vi "multi-graph-example-events.-simplevi.vi"() -> ()   [LabVIEW 2017]
panel:
  out "cycle #":i32
  in  "LSI-U CH labels":string[](array[string])
  out "labels S1":string[](array[string])
  in  "log/linear":bool
  in  "stop":bool
  out "Graph1 (4-10K)":cluster{timestamp[], dbl[]}[](graph)
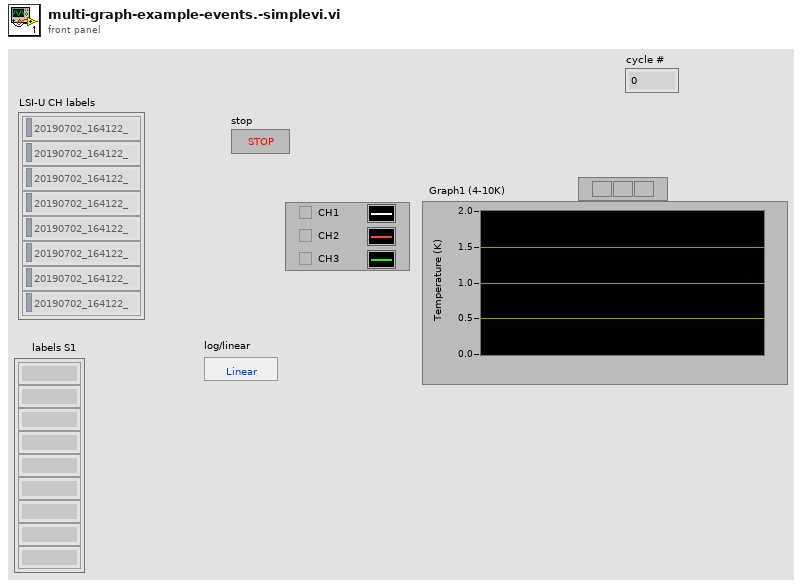
[diagram p1: front panel]
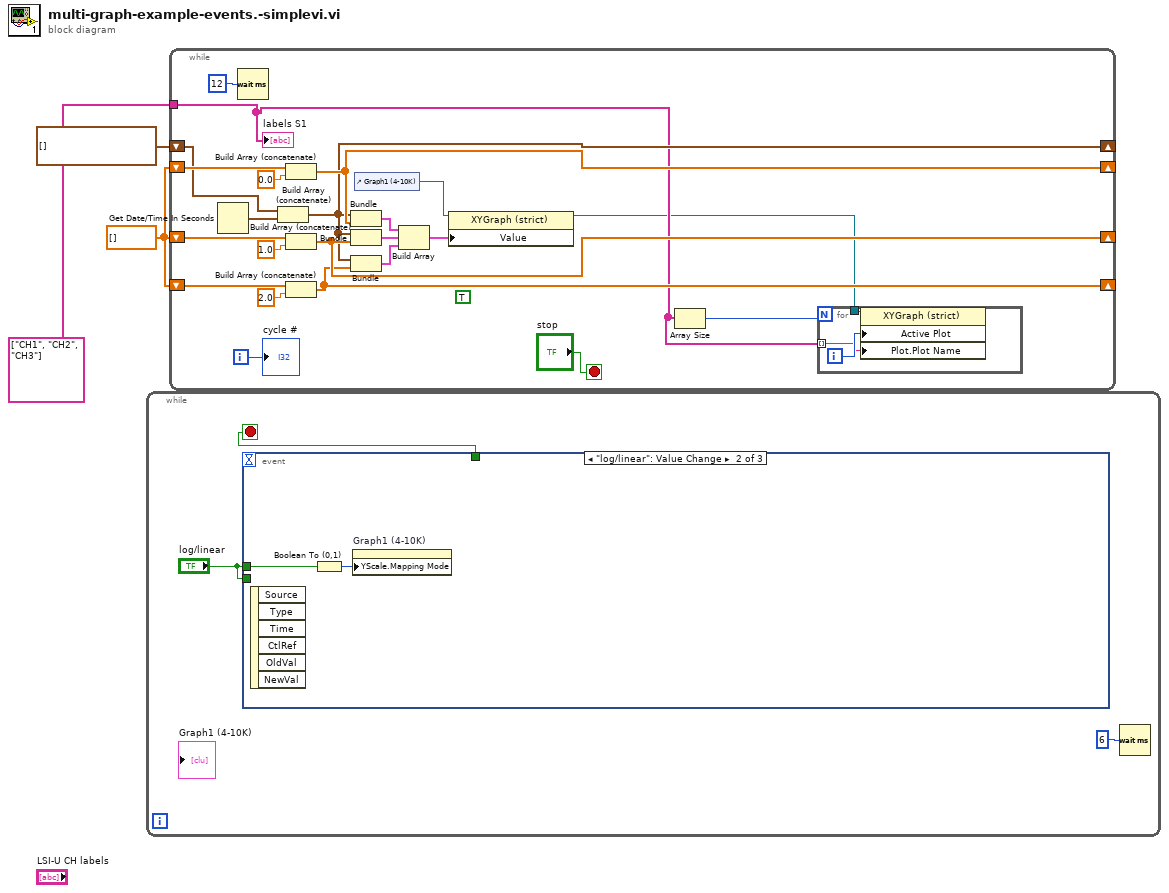
[diagram p0: block diagram]
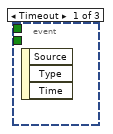
[diagram p2: hidden frame]
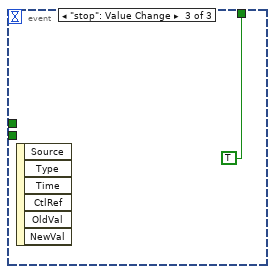
[diagram p3: hidden frame]
diagram:
  w2 = dbl[] []
  n1 = while {
    stop <- w4 stop-if-true
    n2 = event shown="[1] \"log/linear\": Value Change" {
      selector: _ -> [_ _ _]
      dyn-events: _ -> [_ _ _]
      timeout: _ -> [_ _ _]
      tunnel: "log/linear" -> [_ _ _]
      tunnel: "log/linear" -> [_ w7 _]
      tunnel: [_ _ TRUE] -> w4
      event Timeout {
        n3 = event-data() -> ()  [unwired: 1 in, 3 out]
      }
      event "log/linear": Value Change {
        n4 = event-data() -> ()  [unwired: 1 in, 6 out]
        n5 = Boolean To (0,1)(Boolean=w7) -> (0, 1=w8:i16)
        n6 = property on="Graph1 (4-10K)" class="XYGraph (strict)"("YScale.Mapping Mode"=w8) -> ()  [unwired: 2 in, 2 out]
      }
      event "stop": Value Change {
        n7 = event-data() -> ()  [unwired: 1 in, 6 out]
      }
    }
    n8 = Wait (ms)(milliseconds to wait=u32 6) -> ()  [unwired: 1 out]
  }
  n9 = while {
    shift-right: [w26] -> _
    shift-left: w2 -> [w31]
    shift-right: [w20] -> _
    shift-left: timestamp[] [] -> [w29]
    shift-right: [w23] -> _
    shift-left: w2 -> [w24]
    shift-right: [w19] -> _
    shift-left: w2 -> [w21]
    tunnel: string[] ["CH1", "CH2", "CH3"] ("labels S1 2") -> [w11]
    i -> [w15]
    stop <- "stop" stop-if-true
    (unwired) TRUE ("Visible")
    n10 = Get Date/Time In Seconds() -> (seconds since 1Jan1904=w30:timestamp)
    n11 = Wait (ms)(milliseconds to wait=u32 12) -> ()  [unwired: 1 out]
    n12 = Build Array (concatenate)(w29, w30) -> (w20:timestamp[])
    n13 = Build Array (concatenate)(w31, 0.0) -> (w26:dbl[])
    n14 = Build Array (concatenate)(w24, 1.0) -> (w23:dbl[])
    n15 = Build Array (concatenate)(w21, 2.0) -> (w19:dbl[])
    n16 = Bundle(w20, w26) -> (w18:cluster{timestamp[], dbl[]})  [unwired: 1 in]
    n17 = Bundle(w20, w23) -> (w17:cluster{timestamp[], dbl[]})  [unwired: 1 in]
    n18 = Bundle(w20, w19) -> (w16:cluster{timestamp[], dbl[]})  [unwired: 1 in]
    n19 = control-ref of="Graph1 (4-10K)"() -> (w14:refnum<vi>)
    n20 = Build Array(w18, w17, w16) -> (w13:cluster{timestamp[], dbl[]}[])
    n21 = property class="XYGraph (strict)"(reference=w14, "Value"=w13) -> (reference out=w10:refnum<vi>)  [unwired: 1 in, 1 out]
    n22 = Array Size(array=w11) -> (size(s)=w12:i32)
    n23 = for {
      N: w12 -> [_]
      tunnel: w11 -> [w34] mode=indexing
      tunnel: w10 -> [w33]
      i -> [w35]
      n24 = property class="XYGraph (strict)"(reference=w33, "Active Plot"=w35, "Plot.Plot Name"=w34) -> ()  [unwired: 1 in, 2 out]
    }
    "labels S1" <- w11
    "cycle #" <- w15
  }
